vi "Error Handle_Error Info insert Queue.vi"(8 "error in":errorcluster caption="错误输入（无错误）", 11 "error info in":string) -> (0 "error out":errorcluster caption="错误输出")   [LabVIEW 2016]
uses:
  Architecture/Queue Management/ARC_Queue Insert Element.vi
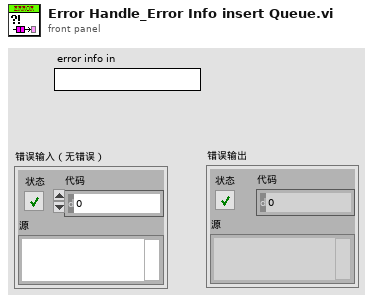
[diagram p1: front panel]
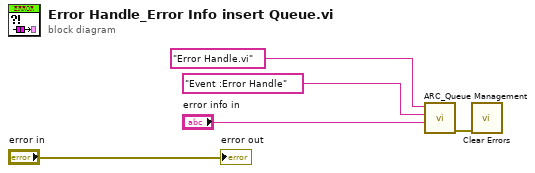
[diagram p0: block diagram]
diagram:
  n1 = call-poly "ARC_Queue Management.vi"("Data"="error info in", "Event"="Event :Error Handle" ("Queue Name(unamed)"), "Queue Name(unamed)"="Error Handle.vi") -> ("error out"=w2:errorcluster)  [unwired: 7 in, 1 out]
  n2 = call <vilib>:"Clear Errors.vi"("error in (no error)"=w2) -> ()  [unwired: 5 in, 2 out]
  "error out" <- "error in"
